vi "niFpgaFFTSimModelCoreWrapper.vi"(0 "real data in":fxp<+/-,16,1>, 1 "reset":bool, 5 "imaginary data in":fxp<+/-,16,1>, 7 "input valid":bool=TRUE, 12 "ready for output":bool=TRUE) -> (3 "data index":u16, 4 "real data out":fxp<+/-,32,16> format="%.21g", 6 "imaginary data out":fxp<+/-,32,16> format="%.21g", 8 "output valid":bool, 14 "ready for input":bool)   [LabVIEW 2017]
uses:
  <vilib>/rvi/Analysis/measure/FFT/simModelSupport/niFPGA FFT Sim Properties.ctl
  <vilib>/rvi/Analysis/measure/FFT/simModelSupport/niFPGA FFT Sim Types.ctl
  <vilib>/rvi/Analysis/measure/FFT/simModelSupport/niFpgaFFTSimArithmeticProperties.ctl
  <vilib>/rvi/Analysis/measure/FFT/simModelSupport/niFpgaFFTSimDfxp.ctl
  <vilib>/fxp/LVFixedPointQuantizationPolicyTypeDef.ctl
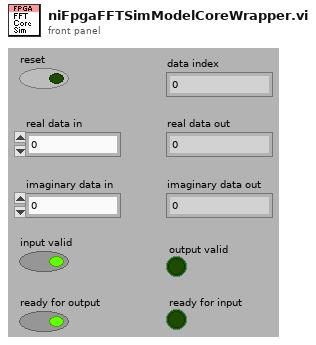
[diagram p1: front panel]
types:
  T1 = typedef "niFPGA FFT Sim Properties.ctl" = cluster{"number of stages":u8, "twiddle over 16?":bool, "forward":bool, "butterfly delay":u16, "N/2":u16, "scale factor":i32, "add control logic register":bool, "Execution Constants":cluster{"N/2-1":u16, "(N/2)*K + 2":u16, "(N/2)*(K-1)+2":u16, "(N/2)*K + 1 + N/2":u16, "N-1":u16, "total latency":u16, "K - 1":u8, "K - 16":i8, "K - 17":i8}, "switch delay":u16, "FFT fxp types":T2}
  T2 = typedef "niFPGA FFT Sim Types.ctl" = cluster{"mult output type":T3, "internal type":T3, "twid type":T3, "sub output type":T3}
  T3 = typedef "niFpgaFFTSimArithmeticProperties.ctl" = cluster{"Output Type":T4, "Adapt To Source?":bool, "Rounding Mode":T5}
  T4 = typedef "niFpgaFFTSimDfxp.ctl" = cluster{"U64 Rep":u64, "Signed?":bool, "Word Length":i32, "Integer Word Length":i32}
  T5 = typedef "LVFixedPointQuantizationPolicyTypeDef.ctl" = enum32{"Truncate", "Round-Half-Up (Asymmetric)", "Round-Half-Even"}
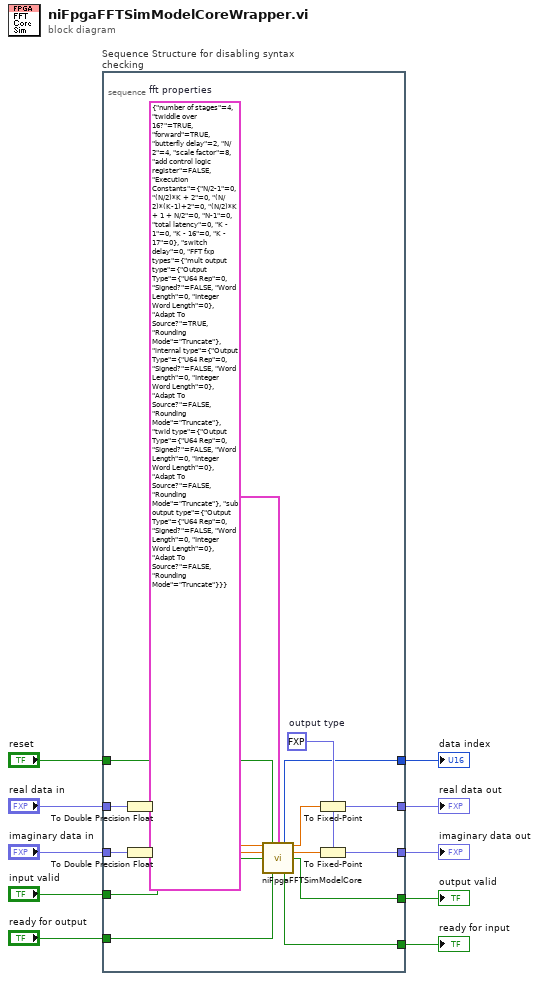
[diagram p0: block diagram]
diagram:
  n1 = stacked-sequence "Sequence Structure for disabling syntax checking" {
    tunnel: "reset" -> [w20]
    tunnel: "real data in" -> [w19]
    tunnel: "imaginary data in" -> [w18]
    tunnel: "input valid" -> [w17]
    tunnel: "ready for output" -> [w16]
    tunnel: [w15] -> w5
    tunnel: [w14] -> w4
    tunnel: [w13] -> w3
    tunnel: [w12] -> w2
    tunnel: [w11] -> w1
    frame #0 {
      w25 = fxp<+/-,32,16> 0.0  # output type
      w26 = T1 {"number of stages"=4, "twiddle over 16?"=TRUE, "forward"=TRUE, "butterfly delay"=2, "N/2"=4, "scale factor"=8, "add control logic register"=FALSE, "Execution Constants"={"N/2-1"=0, "(N/2)*K + 2"=0, "(N/2)*(K-1)+2"=0, "(N/2)*K + 1 + N/2"=0, "N-1"=0, "total latency"=0, "K - 1"=0, "K - 16"=0, "K - 17"=0}, "switch delay"=0, "FFT fxp types"={"mult output type"={"Output Type"={"U64 Rep"=0, "Signed?"=FALSE, "Word Length"=0, "Integer Word Length"=0}, "Adapt To Source?"=TRUE, "Rounding Mode"=enum."Truncate"}, "internal type"={"Output Type"={"U64 Rep"=0, "Signed?"=FALSE, "Word Length"=0, "Integer Word Length"=0}, "Adapt To Source?"=FALSE, "Rounding Mode"=enum."Truncate"}, "twid type"={"Output Type"={"U64 Rep"=0, "Signed?"=FALSE, "Word Length"=0, "Integer Word Length"=0}, "Adapt To Source?"=FALSE, "Rounding Mode"=enum."Truncate"}, "sub output type"={"Output Type"={"U64 Rep"=0, "Signed?"=FALSE, "Word Length"=0, "Integer Word Length"=0}, "Adapt To Source?"=FALSE, "Rounding Mode"=enum."Truncate"}}}  # fft properties
      n2 = To Double Precision Float(number=w19) -> (double precision float=w22:dbl)
      n3 = To Double Precision Float(number=w18) -> (double precision float=w21:dbl)
      n4 = call <vilib>:"niFpgaFFTSimModelCore.vi"("real data in"=w22, "reset"=w20, "input cluster"=w26, "imaginary data in"=w21, "input valid"=w17, "ready for output"=w16) -> ("data index"=w15:u16, "real data out"=w23:dbl, "imaginary data out"=w24:dbl, "output valid"=w12:bool, "ready for input"=w11:bool)  [unwired: 5 out]
      n5 = To Fixed-Point(fixed-point type=w25, number=w23) -> (fixed-point=w14:fxp<+/-,32,16>)
      n6 = To Fixed-Point(fixed-point type=w25, number=w24) -> (fixed-point=w13:fxp<+/-,32,16>)
    }
  }
  "ready for input" <- w1
  "output valid" <- w2
  "real data out" <- w4
  "imaginary data out" <- w3
  "data index" <- w5
